vi "averageSD.vi"(1 "Kinetics in":cluster{"timedelay":dbl[], dbl[]}[](array[cluster])) -> (0 "Kinetics out":cluster{"timedelay":dbl[], dbl[]}[](array[cluster]))   [LabVIEW 2015]
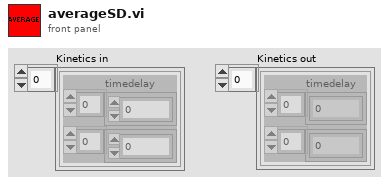
[diagram p1: front panel]
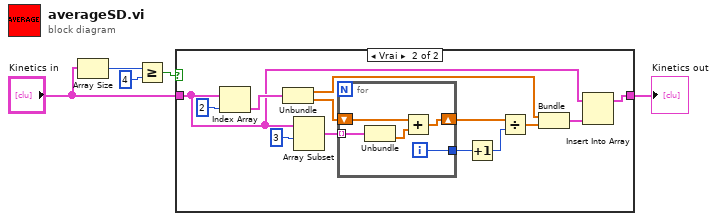
[diagram p0: block diagram]
diagram:
  n1 = Array Size(array="Kinetics in") -> (size(s)=w1:i32)
  n2 = Greater Or Equal?(x=w1, y=4) -> (x >= y?=w3:bool)
  n3 = case shown="Vrai" w3 {
    tunnel: [w6 w14] -> w5
    tunnel: "Kinetics in" -> [w6 w15]
    frame False {
    }
    frame True {
      n4 = Index Array(array=w15, index=2) -> (element=w16:cluster{"timedelay":dbl[], dbl[]})
      n5 = Unbundle(w16) -> ("timedelay"=w12:dbl[], w13:dbl[])
      n6 = Array Subset(array=w15, index=3) -> (w18:cluster{"timedelay":dbl[], dbl[]}[])  [unwired: 1 in]
      n7 = for {
        tunnel: w18 -> [w24] mode=indexing
        shift-right: [w21] -> w10
        shift-left: w13 -> [w23]
        tunnel: [w20] -> w8
        i -> [w20]
        n8 = Unbundle(w24) -> (w22:dbl[])  [unwired: 1 out]
        n9 = Add(x=w23, y=w22) -> (x+y=w21:dbl[])
      }
      n10 = Increment(x=w8) -> (x+1=w7:i32)
      n11 = Divide(x=w10, y=w7) -> (x/y=w9:dbl[])
      n12 = Bundle("timedelay"=w12, w9) -> (w11:cluster{"timedelay":dbl[], dbl[]})  [unwired: 1 in]
      n13 = Insert Into Array(array=w15, new element=w11) -> (w14:cluster{"timedelay":dbl[], dbl[]}[])  [unwired: 1 in]
    }
  }
  "Kinetics out" <- w5
